vi "Check_For_Errors.vi"(8 "Status/Errors in":refnum<vi>, 11 "error in":errorcluster) -> (0 "Status/Errors out":refnum<vi>, 2 "Status":bool, 3 "error out (no error)":errorcluster)   [LabVIEW 2010]
doc: "Check the error cluster if an error has occurred. If so, the Status/Errors-cluster will be updated with the error together with the current time. In all cases the returned error is \"no error\"."
uses:
  Controls/TabPage_Errors.ctl
panel:
  out "Error 1":errorcluster
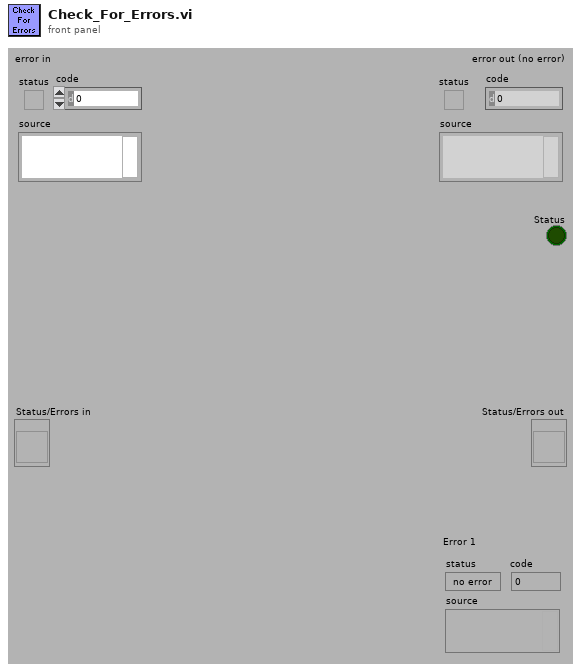
[diagram p1: front panel]
types:
  T1 = typedef "TabPage_Errors.ctl" = cluster{"Errors":string, "Connected?_MAS":bool, "Status_Errors_MAS":bool, "GPS?_MAS":bool, "Slave?_MAS":bool, "Last_Message_MAS":timestamp, "Temperature_MAS":sgl, "Connected?_SLV":bool, "Status_Errors_SLV":bool, "GPS?_SLV":bool, "Slave?_SLV":bool, "Last_Message_SLV":timestamp}
  T2 = typedef "Semaphore RefNum" = refnum<k1>
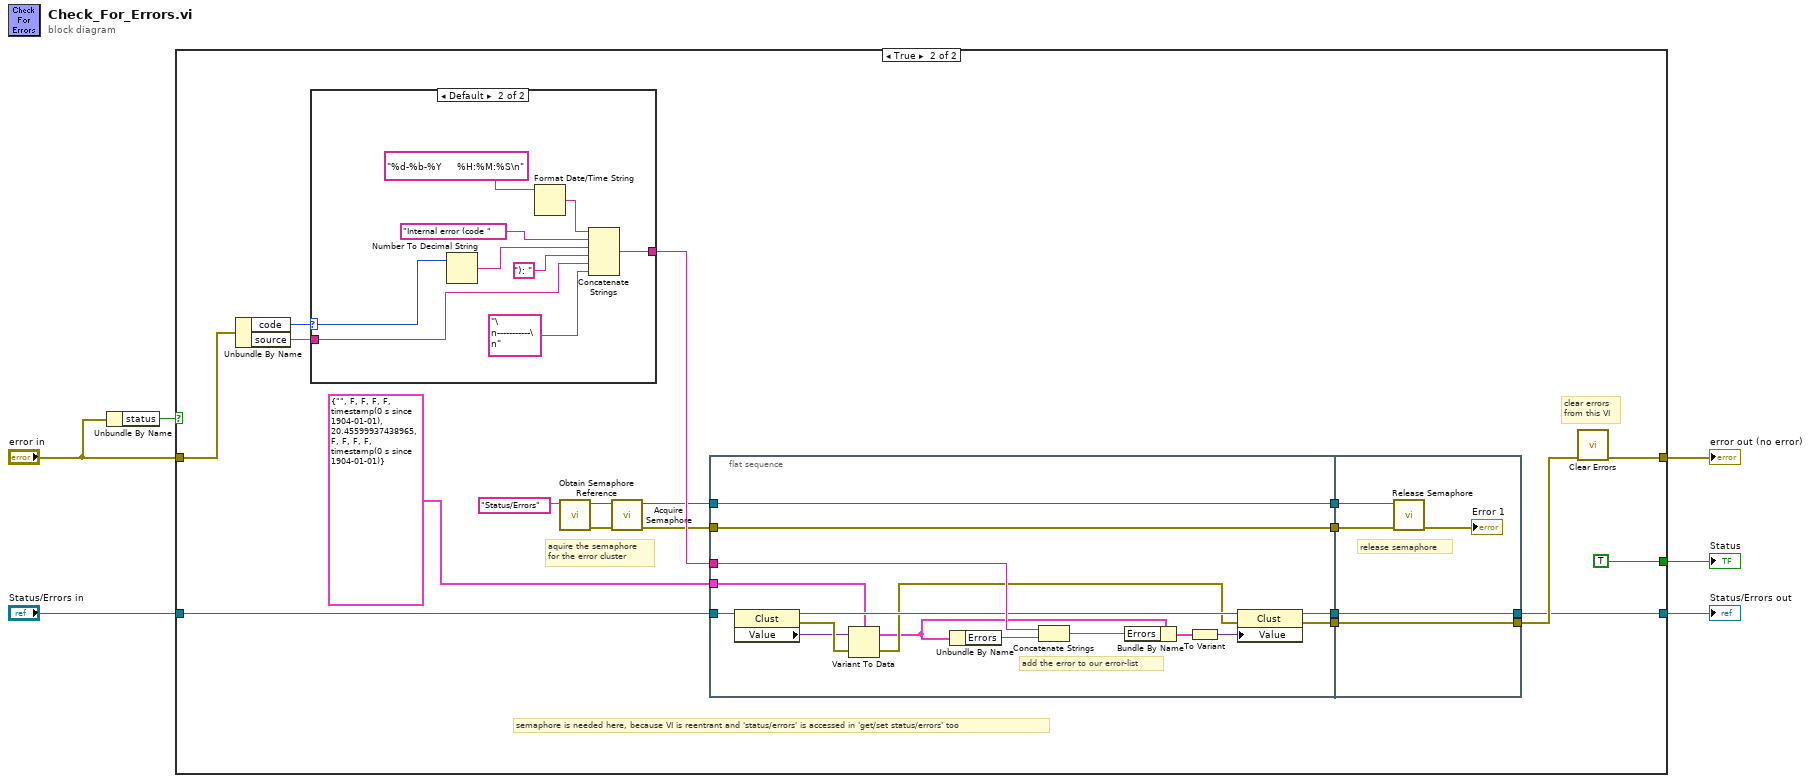
[diagram p0: block diagram]
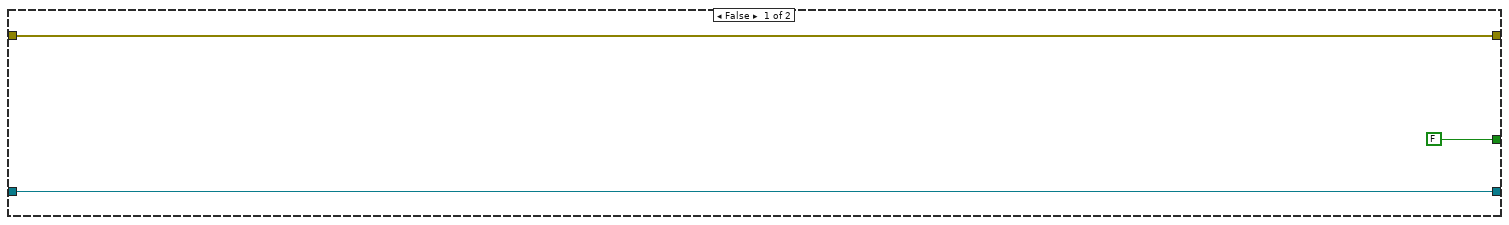
[diagram p2: hidden frame]
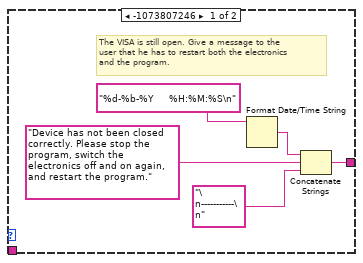
[diagram p3: hidden frame]
diagram:
  n1 = Unbundle By Name("error in") -> ("status"=w2:bool)
  n2 = case shown="True" w2 {
    tunnel: [w8 w19] -> w6
    tunnel: "Status/Errors in" -> [w9 w10]
    tunnel: [w9 w12] -> w4
    tunnel: "error in" -> [w8 w20]
    tunnel: [FALSE TRUE] -> w1
    frame False {
    }
    frame True {
      # "semaphore is needed here, because VI is reentrant and 'status/errors' is accessed in 'get/set status/errors' too"
      # "clear errors\nfrom this VI"
      # "aquire the semaphore\nfor the error cluster"
      n3 = Unbundle By Name(w20) -> ("code"=w24:i32, "source"=w26:string)
      n4 = case shown="Default" w24 {
        selector: w24 -> [_ w55]
        tunnel: [w51 w60] -> w28
        tunnel: w26 -> [_ w59]
        frame -1073807246 {
          # "The VISA is still open. Give a message to the\nuser that he has to restart both the electronics\nand the program."
          n5 = Format Date/Time String(time format string (%c)="%d-%b-%Y     %H:%M:%S\n") -> (date/time string=w53:string)  [unwired: 2 out]
          n6 = Concatenate Strings(w53, "Device has not been closed correctly. Please stop the program, switch the electronics off and on again, and restart the program.", "\n-----------\n") -> (w51:string)
        }
        frame Default {
          n7 = Number To Decimal String(number=w55) -> (decimal integer string=w57:string)  [unwired: 1 out]
          n8 = Format Date/Time String(time format string (%c)="%d-%b-%Y     %H:%M:%S\n") -> (date/time string=w61:string)  [unwired: 2 out]
          n9 = Concatenate Strings(w61, "Internal error (code ", w57, "): ", w59, "\n-----------\n") -> (w60:string)
        }
      }
      n10 = call <vilib>:"Obtain Semaphore Reference.vi"("name (unnamed)"="Status/Errors") -> ("error out"=w23:errorcluster, "semaphore"=w22:T2)  [unwired: 2 in, 3 out]
      n11 = call <vilib>:"Acquire Semaphore.vi"("error in (no error)"=w23, "semaphore"=w22) -> ("error out"=w15:errorcluster, "semaphore out"=w17:T2)  [unwired: 1 in, 3 out]
      n12 = flat-sequence {
        tunnel: w28 -> [w44]
        tunnel: T1 {"Errors"="", "Connected?_MAS"=FALSE, "Status_Errors_MAS"=FALSE, "GPS?_MAS"=FALSE, "Slave?_MAS"=FALSE, "Last_Message_MAS"=timestamp(0 s since 1904-01-01), "Temperature_MAS"=20.456, "Connected?_SLV"=FALSE, "Status_Errors_SLV"=FALSE, "GPS?_SLV"=FALSE, "Slave?_SLV"=FALSE, "Last_Message_SLV"=timestamp(0 s since 1904-01-01)} ("GEN_Page_Statistics") -> [w40]
        tunnel: [w34] -> w18
        tunnel: w17 -> [w34]
        tunnel: [w30] -> w16
        tunnel: w15 -> [w30]
        tunnel: [w33] -> w13
        tunnel: w10 -> [w32]
        tunnel: [w31] -> w11
        tunnel: w18 -> [w49]
        tunnel: w16 -> [w48]
        tunnel: [w46] -> w14
        tunnel: w13 -> [w46]
        tunnel: [w45] -> w12
        tunnel: w11 -> [w45]
        frame #0 {
          # "add the error to our error-list"
          n13 = property class="Clust"(reference=w32) -> (reference out=w41:refnum<vi>, error out=w43:errorcluster, "Value"=w42:variant)  [unwired: 1 in]
          n14 = Variant To Data(error in=w43, Variant=w42, type=w40) -> (error out=w39:errorcluster, data=w38:T1)
          n15 = Unbundle By Name(w38) -> ("Errors"=w35:string)
          n16 = Concatenate Strings(w44, w35) -> (w29:string)
          n17 = Bundle By Name(cluster=w38, "Errors"=w29) -> (w37:T1)
          n18 = To Variant(anything=w37) -> (Variant=w36:variant)
          n19 = property class="Clust"(reference=w41, error in=w39, "Value"=w36) -> (reference out=w31:refnum<vi>, error out=w33:errorcluster)
        }
        frame #1 {
          # "release semaphore"
          n20 = call <vilib>:"Release Semaphore.vi"("error in (no error)"=w48, "semaphore"=w49) -> ("error out"=→"Error 1":errorcluster)  [unwired: 5 out]
        }
      }
      n21 = call <vilib>:"Clear Errors.vi"("error in (no error)"=w14) -> ("error out"=w19:errorcluster)  [unwired: 6 out]
    }
  }
  "error out (no error)" <- w6
  "Status/Errors out" <- w4
  "Status" <- w1
